vi "Z900_navX_Internal_ProcessingLoop.vi"(11 "navX Device":T1={"Interface"={"Protocol"=enum."SERIAL", "Update Rate (4Hz-60Hz)"=4, "navX Open TypeDef"=variant}, "Notify Packet"=refnum, "Loop VI Refnum"=refnum, "Ready to Close Occurrence Refnum"=refnum} {"Interface"."Update Rate (4Hz-60Hz)" min=4 max=60 step=1}) -> (0 "error out":errorcluster, 2 "Registry":u8[](array[numeric]))   [LabVIEW 2015, in "navX Library v2.lvlib"]
doc: "This navX VI handles the reading/writing for the navX. All of the good stuff is in here.\nTHIS VI SHOULD NOT BE CALLED BY THE USER!"
uses:
  navX Library v2.lvlib
  TypeDefs/Z900_navX_DeviceTypeDef.ctl
  TypeDefs/Z900_navX_ProtocolTypeDef.ctl
  TypeDefs/Z900_navX_NotifyPacketTypeDef.ctl
  TypeDefs/Z900_navX_ActionTypeDef.ctl
  <vilib>/Platform/TimedLoop/XDataNode/timing_clust.ctl
  <vilib>/Platform/TimedLoop/XDataNode/nitl_modes.ctl
  <vilib>/Platform/TimedLoop/XDataNode/wakeup.ctl
  TypeDefs/navX Open TypeDefs/Z900_navX_OpenTypeDef_Serial.ctl
  NI WPI/WPI_SerialPort_USB.ctl
  TypeDefs/Z900_navX_SerialStreamTypeDef.ctl
  TypeDefs/Z900_navX_ZeroVectorTypeDef.ctl
  TypeDefs/Z900_navX_DeviceRegisters.ctl
  TypeDefs/Flags/Z900_navX_Flags_CapabilityTypeDef.ctl
  <vilib>/Rock Robotics/SystemInterfaces/Utilities/FPGA_UtilitiesRead LocalTime.vi
  <vilib>/Platform/TimedLoop/XDataNode/XDataNode.xnode
  <vilib>/Platform/TimedLoop/XDataNode/XDNodeRunTimeDep.lvlib
  NI WPI/NI WPI Serial USB.lvlib
panel:
  out "Connected":bool
  in  "Halt":bool
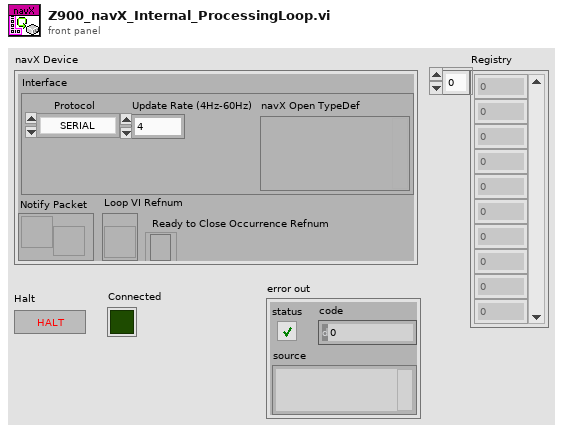
[diagram p1: front panel]
types:
  T1 = typedef "navX Library v2.lvlib/Z900_navX_DeviceTypeDef.ctl" = cluster{"Interface":cluster{"Protocol":T2, "Update Rate (4Hz-60Hz)":u8, "navX Open TypeDef":variant}, "Notify Packet":refnum<notifier>, "Loop VI Refnum":refnum<vi>, "Ready to Close Occurrence Refnum":refnum<k4>}
  T2 = typedef "navX Library v2.lvlib/Z900_navX_ProtocolTypeDef.ctl" = enum16{"SERIAL", "I2C", "SPI"}
  T3 = typedef "navX Library v2.lvlib/Z900_navX_InterfaceTypeDef.ctl" = cluster{"SerialPortRef":T4, "I2CDevRef":T5, "SPIDevRef":T7}
  T4 = typedef "WPI_SerialPortRef.ctl" = cluster{"DevStatus":errorcluster, "Serial Port Name":refnum<visa-resource-name>}
  T5 = typedef "WPI_I2CDevRef.ctl" = cluster{"DevStatus":errorcluster, "Device Address":u8, "Handle":i32, "I2C Bus":T6}
  T6 = typedef "i2c_bus.ctl" = enum16{"I2C On-Board", "I2C MXP", "Invalid"}
  T7 = typedef "WPI_SPIDevRef.ctl" = cluster{"DevStatus":errorcluster, "Handle":i32, "SPI Bus":T8}
  T8 = typedef "spi_bus.ctl" = enum16{"SPI On-Board, CS0", "SPI On-Board, CS1", "SPI On-Board, CS2", "SPI On-Board, CS3", "SPI MXP", "Invalid"}
  T9 = cluster{"Last Valid FPGA Time":dbl, "Error Count":i32, "Initialized":bool}
  T10 = typedef "XDNodeRunTimeDep.lvlib/timing_clust.ctl" = cluster{"Expected End [f-1]":u64, "Actual End [f-1]":u64, "Finished Late? [f-1]":bool, "Expected End [i-1]":u64, "Actual End [i-1]":u64, "Finished Late? [i-1]":bool, "Expected Start [i]":u64, "Actual Start [i]":u64, "Expected Start [f]":u64, "Actual Start [f]":u64, "Source Name":string, "Structure Name":string, "Period":i64, "Deadline":i64, "Offset":i64, "Start":i64, "Priority":i32, "Timeout":i32, "Mode":T11, "Wakeup Reason":T12, "Error":errorcluster, "Source Type":string, "Secondary Source Type":string, "Global End Time":u64, "Global Start Time":u64, "Frame Duration":u64, "Iteration Duration":u64, "Assigned CPU":i32, "I/O Scan Engine Mode":u32}
  T11 = typedef "XDNodeRunTimeDep.lvlib/nitl_modes.ctl" = enum32{"No Change", "Process missed periods, maintain original phase", "Discard missed periods, maintain original phase", "Process missed periods, ignore original phase", "Discard missed periods, ignore original phase"}
  T12 = typedef "XDNodeRunTimeDep.lvlib/wakeup.ctl" = enum32{"Normal", "Aborted", "Asynchronous wakeup", "Timing source error", "Timed loop error", "Timeout"}
  T13 = typedef "navX Library v2.lvlib/Z900_navX_OpenTypeDef_Serial.ctl" = cluster{"Serial Port":T14, "Stream Type":T15}
  T14 = typedef "NI WPI Serial USB.lvlib/WPI_SerialPort_USB.ctl" = enum16{"Onboard RS-232", "MXP TTL", "USB"}
  T15 = typedef "navX Library v2.lvlib/Z900_navX_SerialStreamTypeDef.ctl" = enum16{"YRPH", "Quaterinons", "Gyro/Raw", "AHRS", "AHRSAndPositioning"}
  T16 = typedef "navX Library v2.lvlib/Z900_navX_ZeroVectorTypeDef.ctl" = cluster{"X":bool, "Y":bool, "Z":bool}
  T17 = typedef "navX Library v2.lvlib/Z900_navX_NotifyPacketTypeDef.ctl" = cluster{"navX Action":T18, "Data":variant}
  T18 = typedef "navX Library v2.lvlib/Z900_navX_ActionTypeDef.ctl" = enum16{"None", "Halt", "Update Serial Protocol", "Zero-Yaw", "Zero-Displacement", "Zero-Velocity"}
  T19 = typedef "navX Library v2.lvlib/Z900_navX_DeviceRegisters.ctl" = u8
  T20 = typedef "navX Library v2.lvlib/Z900_navX_Flags_CapabilityTypeDef.ctl" = u16
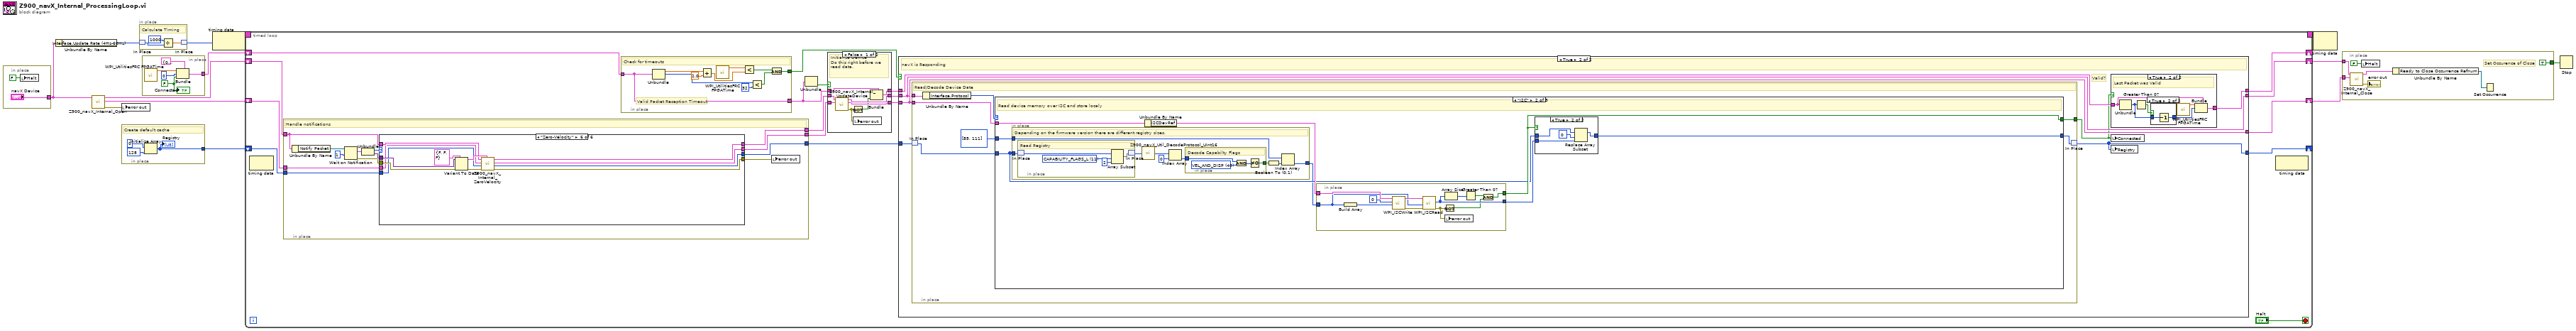
[diagram p0: block diagram]
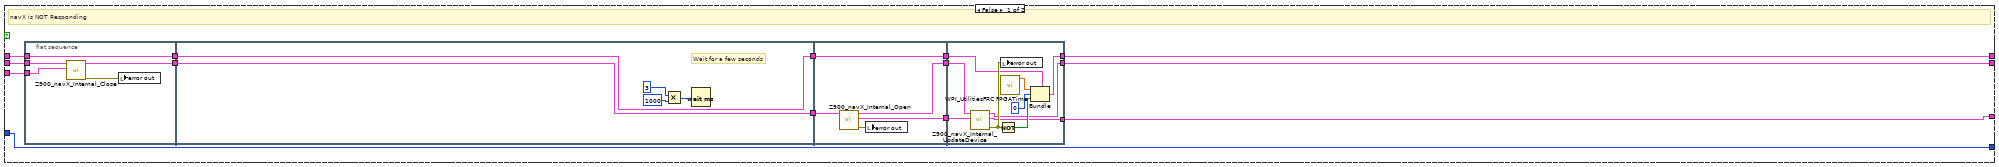
[diagram p3: hidden frame]
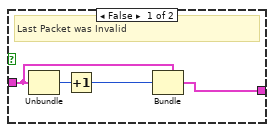
[diagram p4: hidden frame]
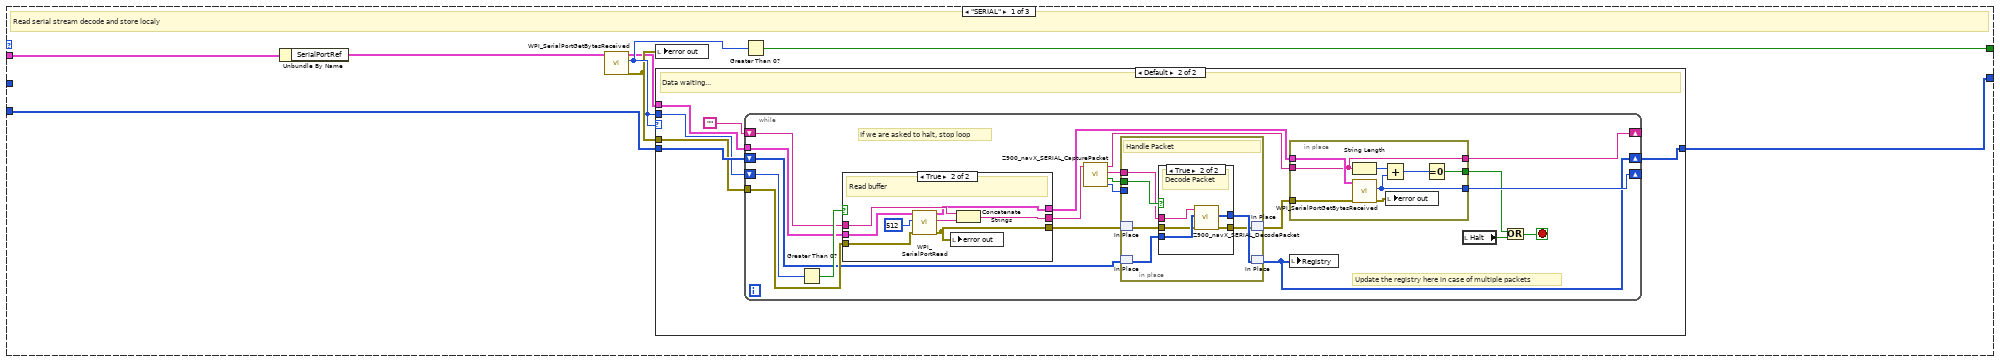
[diagram p6: hidden frame]
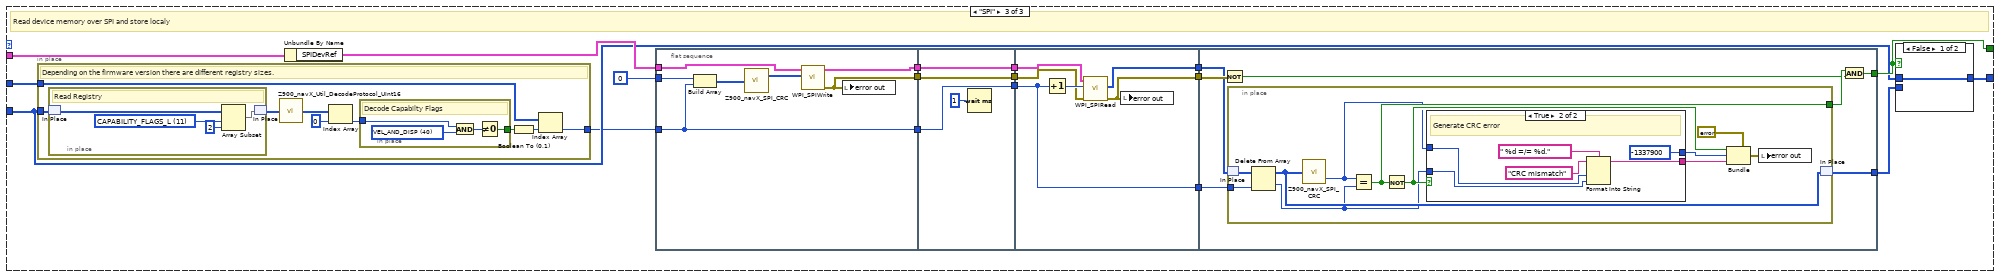
[diagram p11: hidden frame]
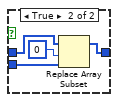
[diagram p12: hidden frame]
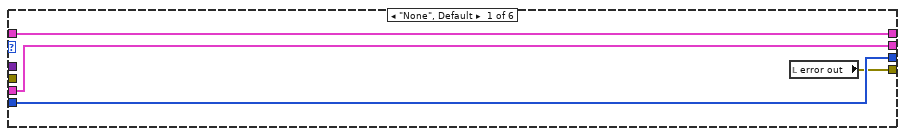
[diagram p14: hidden frame]
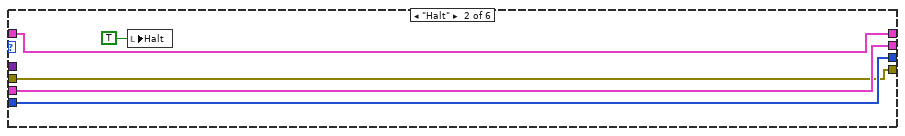
[diagram p15: hidden frame]
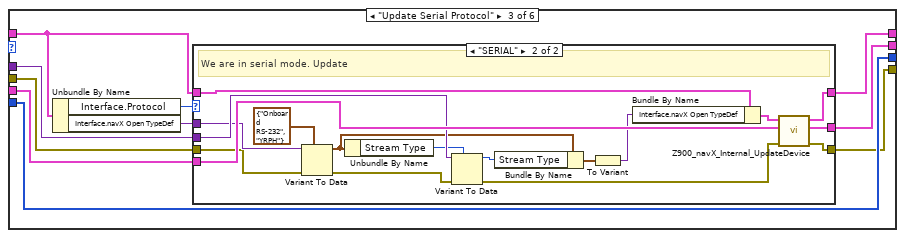
[diagram p16: hidden frame]
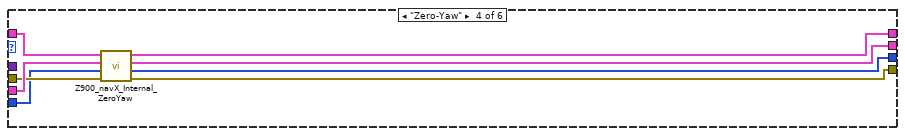
[diagram p18: hidden frame]
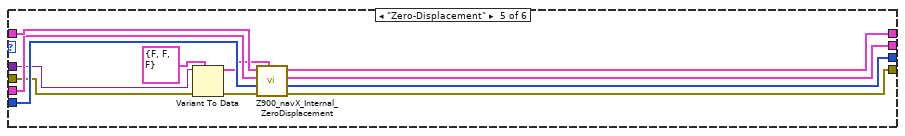
[diagram p19: hidden frame]
diagram:
  n1 = in-place {
    in-place-border: ["navX Device"] -> w6
    n2 = local write "Halt"(FALSE ("Halt")) -> ()
  }
  n3 = Unbundle By Name(w6) -> ("Interface.Update Rate (4Hz-60Hz)"=w10:u8)
  n4 = call "Z900_navX_Internal_Open.vi"("navX Device"=w6) -> ("error out"=w2:errorcluster, "Interface TypeDefs"=w5:T3, "navX Device"=w3:T1)  [unwired: 8 in]
  n5 = local write "error out"(w2) -> ()
  n6 = in-place {
    in-place-border: [w16] -> w9
    # "Create default cache"
    n7 = Initialize Array(u8 0 ("Received Data"), 128 ("hex")) -> (w16:u8[])
    "Registry" <- w16
  }
  n8 = in-place {
    # "Calculate Timing"
    n9 = in-place-match #1(w10) -> (w20:u8)
    n10 = Divide(x=1000, y=w20) -> (x/y=w19:dbl)
    n11 = in-place-match #1(w19) -> (w11:u8)
  }
  n12 = in-place {
    in-place-border: [w24] -> w4
    w22 = FALSE ("Initialized")
    n13 = call <vilib>:"WPI_UtilitiesFRC FPGATime.vi"() -> ("FPGA Time"=w25:dbl)  [unwired: 10 in, 1 out]
    n14 = Bundle(cluster=T9 {"Last Valid FPGA Time"=0.0, "Error Count"=0, "Initialized"=FALSE}, "Last Valid FPGA Time"=w25, "Error Count"=0, "Initialized"=w22) -> (w24:T9)
    "Connected" <- w22
  }
  n15 = node-c288(w11) -> (w13:T10)
  n16 = timed-loop {
    timing: w13 -> [_]
    timing-out: [_] -> w12
    shift-right: [w44] -> _
    shift-left: w9 -> [w39]
    shift-right: [w40] -> w8
    shift-left: w3 -> [w29]
    shift-right: [w42] -> w7
    shift-left: w5 -> [w28]
    shift-right: [w43] -> _
    shift-left: w4 -> [w41]
    stop <- "Halt" stop-if-true
    n17 = node-c288() -> ()  [unwired: 1 in, 1 out]
    n18 = in-place {
      in-place-border: w29 -> [w330]
      in-place-border: w28 -> [w329]
      in-place-border: [w328] -> w32
      in-place-border: [w327] -> w33
      in-place-border: w39 -> [w324]
      in-place-border: [w323] -> w38
      # "Handle notifications"
      n19 = Unbundle By Name(w330) -> ("Notify Packet"=w332:refnum<notifier>)
      n20 = Wait on Notification(notifier=w332, timeout in ms (-1)=1) -> (notification=w334:T17, error out=w325:errorcluster)  [unwired: 2 in, 2 out]
      n21 = Unbundle(w334) -> ("navX Action"=w333:T18, "Data"=w326:variant)
      n22 = case shown="\"Zero-Velocity\"" w333 {
        tunnel: w330 -> [w338 w343 w347 w381 w393 w400]
        tunnel: w329 -> [w337 w342 w353 w379 w391 w399]
        tunnel: [w337 w342 w352 w378 w389 w396] -> w328
        tunnel: [w338 w343 w351 w380 w390 w397] -> w327
        tunnel: w326 -> [_ _ w350 _ w386 w403]
        tunnel: w325 -> [_ w340 w348 w377 w383 w404]
        tunnel: w324 -> [w336 w341 w346 w376 w392 w398]
        tunnel: [w336 w341 w346 w375 w388 w395] -> w323
        tunnel: [w335 w340 w345 w374 w387 w394] -> w322
        frame "None", Default {
          n23 = local read "error out"() -> (w335:errorcluster)
        }
        frame "Halt" {
          n24 = local write "Halt"(TRUE) -> ()
        }
        frame "Update Serial Protocol" {
          n25 = Unbundle By Name(w347) -> ("Interface.Protocol"=w344:T2, "Interface.navX Open TypeDef"=w349:variant)
          n26 = case shown="\"SERIAL\"" w344 {
            tunnel: w353 -> [w355 w373]
            tunnel: [w355 w372] -> w352
            tunnel: [w356 w371] -> w351
            tunnel: w350 -> [_ w370]
            tunnel: w349 -> [_ w367]
            tunnel: w348 -> [w354 w364]
            tunnel: w347 -> [w356 w363]
            tunnel: [w354 w357] -> w345
            frame Default {
              # "We don't care if we are not in serial mode."
            }
            frame "SERIAL" {
              # "We are in serial mode. Update"
              n27 = Variant To Data(error in=w364, type=T13 {"Serial Port"=enum."Onboard RS-232", "Stream Type"=enum."YRPH"} ("navX Serial Open"), Variant=w367) -> (data=w360:T13, error out=w365:errorcluster)
              n28 = Unbundle By Name(w360) -> ("Stream Type"=w359:T15)
              n29 = Variant To Data(error in=w365, type=w359, Variant=w370) -> (data=w358:T15, error out=w369:errorcluster)
              n30 = Bundle By Name(cluster=w360, "Stream Type"=w358) -> (w368:T13)
              n31 = To Variant(anything=w368) -> (Variant=w362:variant)
              n32 = Bundle By Name(cluster=w363, "Interface.navX Open TypeDef"=w362) -> (w361:T1)
              n33 = call "Z900_navX_Internal_UpdateDevice.vi"("error in (no error)"=w369, "Interface TypeDefs"=w373, "navX Device"=w361) -> ("error out"=w357:errorcluster, "Interface TypeDefs"=w372:T3, "navX Device"=w371:T1)  [unwired: 6 in]
            }
          }
        }
        frame "Zero-Yaw" {
          n34 = call "Z900_navX_Internal_ZeroYaw.vi"("error in (no error)"=w377, "Registry"=w376, "Interface TypeDefs"=w379, "navX Device"=w381) -> ("error out"=w374:errorcluster, "Registry"=w375:u8[], "Interface TypeDefs"=w378:T3, "navX Device"=w380:T1)  [unwired: 4 in]
        }
        frame "Zero-Displacement" {
          n35 = Variant To Data(error in=w383, type=T16 {"X"=FALSE, "Y"=FALSE, "Z"=FALSE} ("Zero Vector"), Variant=w386) -> (data=w384:T16, error out=w382:errorcluster)
          n36 = call "Z900_navX_Internal_ZeroDisplacement.vi"("Zero Vector"=w384, "error in (no error)"=w382, "Registry"=w392, "Interface TypeDefs"=w391, "navX Device"=w393) -> ("error out"=w387:errorcluster, "Registry"=w388:u8[], "Interface TypeDefs"=w389:T3, "navX Device"=w390:T1)  [unwired: 3 in]
        }
        frame "Zero-Velocity" {
          n37 = Variant To Data(error in=w404, type=T16 {"X"=FALSE, "Y"=FALSE, "Z"=FALSE} ("Zero Vector"), Variant=w403) -> (data=w402:T16, error out=w401:errorcluster)
          n38 = call "Z900_navX_Internal_ZeroVelocity.vi"("Zero Vector"=w402, "error in (no error)"=w401, "Registry"=w398, "Interface TypeDefs"=w399, "navX Device"=w400) -> ("error out"=w394:errorcluster, "Registry"=w395:u8[], "Interface TypeDefs"=w396:T3, "navX Device"=w397:T1)  [unwired: 3 in]
        }
      }
      n39 = local write "error out"(w322) -> ()
    }
    n40 = in-place {
      in-place-border: w41 -> [w56]
      in-place-border: [w57] -> w37
      in-place-border: [w56] -> w27
      # "Valid Packet Reception Timeout"
      # "Check for timeouts"
      n41 = Unbundle(w56) -> ("Last Valid FPGA Time"=w65:dbl, "Error Count"=w61:i32)  [unwired: 1 out]
      n42 = Add(x=w65, y=2.0) -> (x+y=w63:dbl)
      n43 = call <vilib>:"WPI_UtilitiesFRC FPGATime.vi"() -> ("FPGA Time"=w62:dbl)  [unwired: 10 in, 1 out]
      n44 = Less?(x=w62, y=w63) -> (x < y?=w59:bool)
      n45 = Less?(x=w61, y=32) -> (x < y?=w58:bool)
      n46 = And(x=w59, y=w58) -> (x .and. y?=w57:bool)
    }
    n47 = Unbundle(w27) -> ("Initialized"=w35:bool)  [unwired: 2 out]
    n48 = case shown="False" w35 {
      tunnel: w27 -> [w52 w55]
      tunnel: [w51 w55] -> w34
      tunnel: w33 -> [w50 w54]
      tunnel: w32 -> [w49 w53]
      tunnel: [w48 w54] -> w30
      tunnel: [w47 w53] -> w31
      frame False {
        # "Initialize Device\nDo this right before we\nread data."
        n49 = call "Z900_navX_Internal_UpdateDevice.vi"("Interface TypeDefs"=w49, "navX Device"=w50) -> ("error out"=w46:errorcluster, "Interface TypeDefs"=w47:T3, "navX Device"=w48:T1)  [unwired: 7 in]
        n50 = Not(x=w46) -> (.not. x?=w45:bool)
        n51 = local write "error out"(w46) -> ()
        n52 = Bundle(cluster=w52, "Initialized"=w45) -> (w51:T9)  [unwired: 2 in]
      }
      frame True {
      }
    }
    n53 = case shown="True" w37 {
      tunnel: w38 -> [w77 w111]
      tunnel: w31 -> [w78 w110]
      tunnel: [w77 w107] -> w44
      tunnel: w34 -> [w66 w109]
      tunnel: [w70 w108] -> w43
      tunnel: w30 -> [w79 w106]
      tunnel: [w71 w106] -> w40
      tunnel: [w74 w110] -> w42
      frame False {
        # "navX is NOT Responding"
        n54 = flat-sequence {
          tunnel: w79 -> [w82]
          tunnel: w78 -> [w84]
          tunnel: [w83] -> w76
          tunnel: [w80] -> w67
          tunnel: w66 -> [w80]
          tunnel: w76 -> [w89]
          tunnel: [w89] -> w75
          tunnel: [w85] -> w68
          tunnel: w67 -> [w85]
          tunnel: w75 -> [w93]
          tunnel: [w94] -> w73
          tunnel: [w92] -> w72
          tunnel: [w90] -> w69
          tunnel: w68 -> [w90]
          tunnel: [w102] -> w70
          tunnel: [w98] -> w74
          tunnel: [w99] -> w71
          tunnel: w69 -> [w97]
          tunnel: w72 -> [w100]
          tunnel: w73 -> [w101]
          frame #0 {
            n55 = call "Z900_navX_Internal_Close.vi"("Interface TypeDefs"=w84, "navX Device"=w82) -> ("error out"=w81:errorcluster, "navX Device"=w83:T1)  [unwired: 8 in]
            n56 = local write "error out"(w81) -> ()
          }
          frame #1 {
            # "Wait for a few seconds"
            n57 = Multiply(x=u32 3 ("milliseconds to wait"), y=u32 1000) -> (x*y=w87:u32)
            n58 = Wait (ms)(milliseconds to wait=w87) -> ()  [unwired: 1 out]
          }
          frame #2 {
            n59 = call "Z900_navX_Internal_Open.vi"("navX Device"=w93) -> ("error out"=w91:errorcluster, "Interface TypeDefs"=w92:T3, "navX Device"=w94:T1)  [unwired: 8 in]
            n60 = local write "error out"(w91) -> ()
          }
          frame #3 {
            n61 = call "Z900_navX_Internal_UpdateDevice.vi"("Interface TypeDefs"=w100, "navX Device"=w101) -> ("error out"=w103:errorcluster, "Interface TypeDefs"=w98:T3, "navX Device"=w99:T1)  [unwired: 7 in]
            n62 = Not(x=w103) -> (.not. x?=w104:bool)
            n63 = local write "error out"(w103) -> ()
            n64 = call <vilib>:"WPI_UtilitiesFRC FPGATime.vi"() -> ("FPGA Time"=w96:dbl)  [unwired: 10 in, 1 out]
            n65 = Bundle(cluster=w97, "Last Valid FPGA Time"=w96, "Error Count"=0, "Initialized"=w104) -> (w102:T9)
          }
        }
      }
      frame True {
        # "Valid?"
        # "navX is Responding"
        n66 = in-place {
          in-place-border: w106 -> [w126]
          in-place-border: w110 -> [w130]
          in-place-border: [w128] -> w105
          # "Read/Decode Device Date"
          n67 = in-place-match #2(w111) -> (w129:u8[])
          n68 = Unbundle By Name(w126) -> ("Interface.Protocol"=w131:T2)
          n69 = case shown="\"I2C\"" w131 {
            tunnel: [w137 w204 w251] -> w127
            tunnel: w129 -> [w138 w201 w243]
            tunnel: w130 -> [w139 w206 w258]
            tunnel: [w135 w203 w248] -> w128
            tunnel: i32[] [85, 111] -> [_ w200 w242]
            frame "SERIAL" {
              # "Read serial stream decode and store localy"
              n70 = Unbundle By Name(w139) -> ("SerialPortRef"=w136:T4)
              n71 = call <vilib>:"WPI_SerialPortGetBytesReceived.vi"("SerialPortRef"=w136) -> ("error out"=w133:errorcluster, "Bytes at Port"=w134:u32, "SerialPortRef"=w132:T4)  [unwired: 8 in]
              n72 = local write "error out"(w133) -> ()
              n73 = case shown="Default" w134 {
                tunnel: [w140 w146] -> w137
                tunnel: w138 -> [w140 w145]
                tunnel: w134 -> [_ w144]
                tunnel: w132 -> [_ w142]
                tunnel: w133 -> [_ w141]
                frame 0 {
                }
                frame Default {
                  # "Data waiting..."
                  n74 = while {
                    shift-right: [w148] -> w146
                    shift-left: w145 -> [w155]
                    shift-right: [w159] -> _
                    shift-left: w144 -> [w166]
                    shift-right: [w158] -> _
                    shift-left: "" -> [w164]
                    tunnel: w142 -> [w163]
                    tunnel: w141 -> [w162]
                    stop <- w151 stop-if-true
                    # "Update the registry here in case of multiple packets"
                    # "If we are asked to halt, stop loop"
                    n75 = Greater Than 0?(x=w166) -> (x > 0?=w165:bool)
                    n76 = case shown="True" w165 {
                      tunnel: w164 -> [w190 w198]
                      tunnel: w163 -> [w189 w197]
                      tunnel: w162 -> [w188 w194]
                      tunnel: [w190 w193] -> w161
                      tunnel: [w189 w192] -> w147
                      tunnel: [w188 w191] -> w154
                      frame False {
                        # "Pass existing buffer"
                      }
                      frame True {
                        # "Read buffer"
                        n77 = call <vilib>:"WPI_SerialPortRead.vi"("error in (no error)"=w194, "Num Bytes to Read"=u32 512, "SerialPortRef"=w197) -> ("error out"=w191:errorcluster, "Buffer"=w196:string, "SerialPortRef"=w192:T4)  [unwired: 6 in]
                        n78 = local write "error out"(w191) -> ()
                        n79 = Concatenate Strings(w198, w196) -> (w193:string)
                      }
                    }
                    n80 = call "Z900_navX_SERIAL_CapturePacket.vi"("Buffer"=w161) -> ("Packet Size"=w156:i32, "Packet Located"=w149:bool, "Packet"=w157:string, "Buffer"=w160:string)  [unwired: 7 in]
                    n81 = in-place {
                      in-place-border: w157 -> [w171]
                      in-place-border: w149 -> [w172]
                      in-place-border: w156 -> [_]
                      # "Handle Packet"
                      n82 = in-place-match #3(w154) -> (w168:errorcluster)
                      n83 = in-place-match #4(w155) -> (w169:u8[])
                      n84 = case shown="True" w172 {
                        tunnel: w171 -> [_ w179]
                        tunnel: [w174 w177] -> w170
                        tunnel: w169 -> [w174 w178]
                        tunnel: w168 -> [w173 w176]
                        tunnel: [w173 w175] -> w167
                        frame False {
                          # "No Packet"
                        }
                        frame True {
                          # "Decode Packet"
                          n85 = call "Z900_navX_SERIAL_DecodePacket.vi"("error in (no error)"=w176, "Data"=w178, "Packet"=w179) -> ("error out"=w175:errorcluster, "Data"=w177:u8[])  [unwired: 6 in, 1 out]
                        }
                      }
                      n86 = in-place-match #3(w167) -> (w153:errorcluster)
                      n87 = in-place-match #4(w170) -> (w148:u8[])
                    }
                    n88 = in-place {
                      in-place-border: w147 -> [w187]
                      in-place-border: w153 -> [w186]
                      in-place-border: w160 -> [w181]
                      in-place-border: [w183] -> w152
                      in-place-border: [w182] -> w159
                      in-place-border: [w181] -> w158
                      n89 = String Length(string=w181) -> (length=w184:i32)
                      n90 = call <vilib>:"WPI_SerialPortGetBytesReceived.vi"("error in (no error)"=w186, "SerialPortRef"=w187) -> ("error out"=w180:errorcluster, "Bytes at Port"=w182:u32)  [unwired: 7 in, 1 out]
                      n91 = Add(x=w184, y=w182) -> (x+y=w185:u32)
                      n92 = local write "error out"(w180) -> ()
                      n93 = Equal To 0?(x=w185) -> (x = 0?=w183:bool)
                    }
                    n94 = local write "Registry"(w148) -> ()
                    n95 = local read "Halt"() -> (w150:bool)
                    n96 = Or(x=w152, y=w150) -> (x .or. y?=w151:bool)
                  }
                }
              }
              n97 = Greater Than 0?(x=w134) -> (x > 0?=w135:bool)
            }
            frame "I2C" {
              # "Read device memory over I2C and store localy"
              n98 = in-place {
                in-place-border: w201 -> [w215]
                in-place-border: w200 -> [w208]
                in-place-border: [w207] -> w199
                # "Depending on the firmware version there are different registry sizes."
                n99 = in-place {
                  w223 = T19 11 items=["WHOAMI"=0, "HW_REV"=1, "FW_VER_MAJOR"=2, "FW_VER_MINOR"=3, "UPDATE_RATE_HZ"=4, "ACCEL_FSR_G"=5, "GYRO_FSR_DPS"=6, "OP_STATUS"=8, "CAL_STATUS"=9, "SELFTEST_STATUS"=10, "CAPABILITY_FLAGS_L"=11, "CAPABILITY_FLAGS_H"=12, "SENSOR_STATUS"=16, "TIMESTAMP"=18, "YAW"=22, "ROLL"=24, "PITCH"=26, "HEADING"=28, "FUSED_HEADING"=30, "ALTITUDE_I"=32, "ALTITUDE_D"=34, "LINERA_ACC_X"=36, "LINERA_ACC_Y"=38, "LINERA_ACC_Z"=40, "QUAT_W"=42, "QUAT_X"=44, "QUAT_Y"=46, "QUAT_Z"=48, "MPU_TEMP_C"=50, "GYRO_X"=52, "GYRO_Y"=54, "GYRO_Z"=56, "ACC_X"=58, "ACC_Y"=60, "ACC_Z"=62, "MAG_X"=64, "MAG_Y"=66, "MAG_Z"=68, "PRESSURE_I"=70, "PRESSURE_D"=72, "PRESSURE_TEMP"=74, "YAW_OFFSET"=76, "QUAT_OFFSET_W"=78, "QUAT_OFFSET_X"=80, "QUAT_OFFSET_Y"=82, "QUAT_OFFSET_Z"=84, "INTEGRATION_CONTROL"=86, "VELOCITY_X"=88, "VELOCITY_Y"=92, "VELOCITY_Z"=96, "DISPLACMENT_X"=100, "DISPLACMENT_Y"=104, "DISPLACEMENT_Z"=108] ("Device Register")
                  # "Read Registry"
                  n100 = in-place-match #5(w215) -> (w221:u8[])
                  n101 = Array Subset(array=w221, index=w223, length=2) -> (w222:u8[])
                  n102 = in-place-match #5(w222) -> (w212:u8[])
                }
                n103 = call "Z900_navX_Util_DecodeProtocol_UInt16.vi"("Little Endian"=w212) -> ("UInt16"=w213:u16[])
                n104 = Index Array(array=w213, index=0) -> (element=w211:u16)
                n105 = in-place {
                  in-place-border: w211 -> [w217]
                  in-place-border: [w216] -> w210
                  w219 = T20 40 items=["OMNIMOUNT"=4, "OMNIMOUNT_CONFIG_MASK"=38, "VEL_AND_DISP"=40, "YAW_RESET"=80] ("Capability Flag")
                  # "Decode Capabilty Flags"
                  n106 = And(x=w217, y=w219) -> (x .and. y?=w218:T20)
                  n107 = Not Equal To 0?(x=w218) -> (x != 0?=w216:bool)
                }
                n108 = Boolean To (0,1)(Boolean=w210) -> (0, 1=w209:i16)
                n109 = Index Array(array=w208, index=w209) -> (element=w207:i32)
              }
              n110 = Unbundle By Name(w206) -> ("I2CDevRef"=w202:T5)
              n111 = in-place {
                in-place-border: [w229] -> w205
                in-place-border: [w228] -> w203
                in-place-border: w202 -> [w226]
                in-place-border: w199 -> [w224]
                n112 = Build Array(w224) -> (w235:i32[])
                n113 = call <vilib>:"WPI_I2CWrite.vi"("I2CDataToSend"=w235, "I2CRegister"=u8 0 ("hex"), "I2CDevRef"=w226) -> ("error out"=w234:errorcluster, "I2CDevRef"=w233:T5)  [unwired: 7 in]
                n114 = call <vilib>:"WPI_I2CRead.vi"("error in (no error)"=w234, "I2CBytesToRead"=w224, "I2CDevRef"=w233) -> ("error out"=w225:errorcluster, "Data Out"=w229:u8[])  [unwired: 6 in, 1 out]
                n115 = Not(x=w225) -> (.not. x?=w227:bool)
                n116 = Array Size(array=w229) -> (size(s)=w231:i32)
                n117 = local write "error out"(w225) -> ()
                n118 = Greater Than 0?(x=w231) -> (x > 0?=w230:bool)
                n119 = And(x=w230, y=w227) -> (x .and. y?=w228:bool)
              }
              n120 = case shown="True" w203 {
                tunnel: w201 -> [w236 w240]
                tunnel: [w236 w239] -> w204
                tunnel: w205 -> [_ w238]
                frame False {
                }
                frame True {
                  n121 = Replace Array Subset(array=w240, new element=w238, index=u8 0 ("hex")) -> (w239:u8[])
                }
              }
            }
            frame "SPI" {
              # "Read device memory over SPI and store localy"
              n122 = in-place {
                in-place-border: w243 -> [w267]
                in-place-border: w242 -> [w260]
                in-place-border: [w259] -> w241
                # "Depending on the firmware version there are different registry sizes."
                n123 = in-place {
                  w275 = T19 11 items=["WHOAMI"=0, "HW_REV"=1, "FW_VER_MAJOR"=2, "FW_VER_MINOR"=3, "UPDATE_RATE_HZ"=4, "ACCEL_FSR_G"=5, "GYRO_FSR_DPS"=6, "OP_STATUS"=8, "CAL_STATUS"=9, "SELFTEST_STATUS"=10, "CAPABILITY_FLAGS_L"=11, "CAPABILITY_FLAGS_H"=12, "SENSOR_STATUS"=16, "TIMESTAMP"=18, "YAW"=22, "ROLL"=24, "PITCH"=26, "HEADING"=28, "FUSED_HEADING"=30, "ALTITUDE_I"=32, "ALTITUDE_D"=34, "LINERA_ACC_X"=36, "LINERA_ACC_Y"=38, "LINERA_ACC_Z"=40, "QUAT_W"=42, "QUAT_X"=44, "QUAT_Y"=46, "QUAT_Z"=48, "MPU_TEMP_C"=50, "GYRO_X"=52, "GYRO_Y"=54, "GYRO_Z"=56, "ACC_X"=58, "ACC_Y"=60, "ACC_Z"=62, "MAG_X"=64, "MAG_Y"=66, "MAG_Z"=68, "PRESSURE_I"=70, "PRESSURE_D"=72, "PRESSURE_TEMP"=74, "YAW_OFFSET"=76, "QUAT_OFFSET_W"=78, "QUAT_OFFSET_X"=80, "QUAT_OFFSET_Y"=82, "QUAT_OFFSET_Z"=84, "INTEGRATION_CONTROL"=86, "VELOCITY_X"=88, "VELOCITY_Y"=92, "VELOCITY_Z"=96, "DISPLACMENT_X"=100, "DISPLACMENT_Y"=104, "DISPLACEMENT_Z"=108] ("Device Register")
                  # "Read Registry"
                  n124 = in-place-match #6(w267) -> (w273:u8[])
                  n125 = Array Subset(array=w273, index=w275, length=2) -> (w274:u8[])
                  n126 = in-place-match #6(w274) -> (w264:u8[])
                }
                n127 = call "Z900_navX_Util_DecodeProtocol_UInt16.vi"("Little Endian"=w264) -> ("UInt16"=w265:u16[])
                n128 = Index Array(array=w265, index=0) -> (element=w263:u16)
                n129 = in-place {
                  in-place-border: w263 -> [w269]
                  in-place-border: [w268] -> w262
                  w271 = T20 40 items=["OMNIMOUNT"=4, "OMNIMOUNT_CONFIG_MASK"=38, "VEL_AND_DISP"=40, "YAW_RESET"=80] ("Capability Flag")
                  # "Decode Capabilty Flags"
                  n130 = And(x=w269, y=w271) -> (x .and. y?=w270:T20)
                  n131 = Not Equal To 0?(x=w270) -> (x != 0?=w268:bool)
                }
                n132 = Boolean To (0,1)(Boolean=w262) -> (0, 1=w261:i16)
                n133 = Index Array(array=w260, index=w261) -> (element=w259:i32)
              }
              n134 = Unbundle By Name(w258) -> ("SPIDevRef"=w244:T7)
              n135 = flat-sequence {
                tunnel: u8 0 ("hex") -> [w287]
                tunnel: w241 -> [w282]
                tunnel: w244 -> [w284]
                tunnel: [w283] -> w257
                tunnel: [w282] -> w254
                tunnel: [w281] -> w247
                tunnel: w257 -> [w290]
                tunnel: [w290] -> w256
                tunnel: [w289] -> w255
                tunnel: w254 -> [w289]
                tunnel: w247 -> [w288]
                tunnel: [w288] -> w246
                tunnel: w256 -> [w297]
                tunnel: w255 -> [w294]
                tunnel: [w295] -> w253
                tunnel: [w294] -> w252
                tunnel: w246 -> [w293]
                tunnel: [w292] -> w245
                tunnel: w253 -> [w300]
                tunnel: w252 -> [w304]
                tunnel: [w301] -> w248
                tunnel: [w299] -> w250
                tunnel: w245 -> [w303]
                frame #0 {
                  n136 = Build Array(w287, w282) -> (w286:i32[])
                  n137 = call "Z900_navX_SPI_CRC.vi"("Message"=w286) -> ("Message with CRC"=w285:u8[])  [unwired: 1 out]
                  n138 = call <vilib>:"WPI_SPIWrite.vi"("Data To Send"=w285, "SPIDevRef"=w284) -> ("error out"=w281:errorcluster, "SPIDevRef"=w283:T7)  [unwired: 7 in, 1 out]
                  n139 = local write "error out"(w281) -> ()
                }
                frame #1 {
                  n140 = Wait (ms)(milliseconds to wait=u32 1) -> ()  [unwired: 1 out]
                }
                frame #2 {
                  n141 = Increment(x=w294) -> (x+1=w296:i32)
                  n142 = call <vilib>:"WPI_SPIRead.vi"("error in (no error)"=w293, "Num to Read"=w296, "SPIDevRef"=w297) -> ("error out"=w292:errorcluster, "Received Data"=w295:u8[])  [unwired: 6 in, 1 out]
                  n143 = local write "error out"(w292) -> ()
                }
                frame #3 {
                  n144 = Not(x=w303) -> (.not. x?=w298:bool)
                  n145 = in-place {
                    in-place-border: w304 -> [w315]
                    in-place-border: [w312] -> w302
                    n146 = in-place-match #7(w300) -> (w314:u8[])
                    n147 = Delete From Array(array=w314, index=w315) -> (deleted portion=w309:u8, array with subset deleted=w313:u8[])  [unwired: 1 in]
                    n148 = call "Z900_navX_SPI_CRC.vi"("Message"=w313) -> ("CRC"=w310:u8)  [unwired: 1 out]
                    n149 = Equal?(x=w310, y=w309) -> (x = y?=w312:bool)
                    n150 = Not(x=w312) -> (.not. x?=w311:bool)
                    n151 = case shown="True" w311 {
                      tunnel: w310 -> [_ w319]
                      tunnel: w309 -> [_ w318]
                      tunnel: [_ w317] -> w308
                      tunnel: [_ -1337900 ("code")] -> w305
                      frame False {
                      }
                      frame True {
                        # "Generate CRC error"
                        n152 = Format Into String(format string=" %d =/= %d.", initial string="CRC mismatch", w319, w318) -> (resulting string=w317:string)  [unwired: 1 in, 1 out]
                      }
                    }
                    n153 = Bundle(cluster=errorcluster {"status"=FALSE, "code"=0, "source"=""} ("error constant"), "status"=w311, "code"=w305, "source"=w308) -> (w306:errorcluster)
                    n154 = local write "error out"(w306) -> ()
                    n155 = in-place-match #7(w313) -> (w299:u8[])
                  }
                  n156 = And(x=w302, y=w298) -> (x .and. y?=w301:bool)
                }
              }
              n157 = case shown="False" w248 {
                tunnel: w243 -> [w276 w280]
                tunnel: [w276 w279] -> w251
                tunnel: w250 -> [_ w278]
                frame False {
                }
                frame True {
                  n158 = Replace Array Subset(array=w280, new element=w278, index=u8 0 ("hex")) -> (w279:u8[])
                }
              }
            }
          }
          n159 = in-place-match #2(w127) -> (w107:u8[])
        }
        n160 = case shown="True" w105 {
          tunnel: [w112 w120] -> w108
          tunnel: w109 -> [w113 w119]
          frame False {
            # "Last Packet was Invalid"
            n161 = Unbundle(w113) -> ("Error Count"=w114:i32)  [unwired: 2 out]
            n162 = Increment(x=w114) -> (x+1=w115:i32)
            n163 = Bundle(cluster=w113, "Error Count"=w115) -> (w112:T9)  [unwired: 2 in]
          }
          frame True {
            # "Last Packet was Valid"
            n164 = Unbundle(w119) -> ("Error Count"=w117:i32)  [unwired: 2 out]
            n165 = Greater Than 0?(x=w117) -> (x > 0?=w118:bool)
            n166 = case shown="True" w118 {
              tunnel: [w122 w123] -> w116
              tunnel: w117 -> [w122 w124]
              frame False {
              }
              frame True {
                n167 = Decrement(x=w124) -> (x-1=w123:i32)
              }
            }
            n168 = call <vilib>:"WPI_UtilitiesFRC FPGATime.vi"() -> ("FPGA Time"=w121:dbl)  [unwired: 10 in, 1 out]
            n169 = Bundle(cluster=w119, "Last Valid FPGA Time"=w121, "Error Count"=w116) -> (w120:T9)  [unwired: 1 in]
          }
        }
        n170 = local write "Connected"(w105) -> ()
        n171 = local write "Registry"(w107) -> ()
      }
    }
    n172 = node-c288() -> ()  [unwired: 1 in, 1 out]
  }
  n173 = node-c288(w12) -> ()  [unwired: 1 out]
  n174 = in-place {
    in-place-border: w8 -> [w414]
    in-place-border: w7 -> [w413]
    in-place-border: [TRUE] -> w1
    # "Set Occurence of Close"
    n175 = call "Z900_navX_Internal_Close.vi"("Interface TypeDefs"=w413, "navX Device"=w414) -> ("error out"=→"error out":errorcluster, "navX Device"=w408:T1)  [unwired: 8 in]
    n176 = local write "Halt"(FALSE ("Halt")) -> ()
    n177 = Unbundle By Name(w408) -> ("Ready to Close Occurrence Refnum"=w410:refnum<k4>)
    n178 = Set Occurrence(w410) -> ()
  }
  n179 = Stop(stop? (T)=w1) -> ()
